vi "UnicodeArrayToAsciiString.vi"(11 "In array":u8[](array[numeric])) -> (3 "String":string)   [LabVIEW 2019]
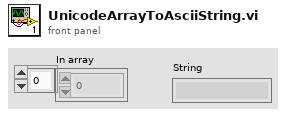
[diagram p1: front panel]
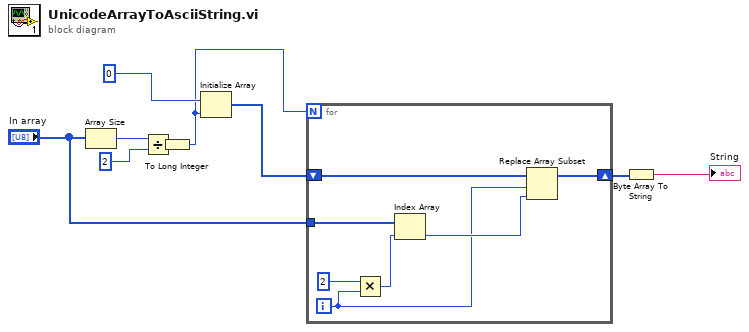
[diagram p0: block diagram]
diagram:
  n1 = Array Size(array="In array") -> (size(s)=w6:i32)
  n2 = Divide(x=w6, y=2) -> (x/y=w8:dbl)
  n3 = To Long Integer(number=w8) -> (32bit integer=w3:i32)
  n4 = Initialize Array(u8 0, w3) -> (w5:u8[])
  n5 = for {
    N: w3 -> [_]
    shift-right: [w16] -> w2
    shift-left: w5 -> [w10]
    tunnel: "In array" -> [w14]
    i -> [w11]
    n6 = Multiply(x=2, y=w11) -> (x*y=w13:i32)
    n7 = Index Array(array=w14, index=w13) -> (element=w12:u8)
    n8 = Replace Array Subset(array=w10, new element=w12, index=w11) -> (w16:u8[])
  }
  n9 = Byte Array To String(unsigned byte array=w2) -> (string=→"String":string)
